vi "Read Device Info.vi"(8 "Error In":errorcluster, 11 "AMS Connection In":T3) -> (0 "Error Out":errorcluster, 1 "Version":T2, 2 "ADS Error":T1 items=["NoError"=0, "InternalError"=1, "NoRTime"=2, "LockedMemoryError"=3, "MailBoxError"=4, "WrongHMsg"=5, "TargetPortNotFound"=6, "TargetMachineNotFound"=7, "UnknownCommandID"=8, "BadTaskID"=9, "NoIO"=10, "UnknownAmsCommand"=11, "Win32Error"=12, "PortNotConnected"=13, "InvalidAmsLength"=14, "InvalidAmsNetID"=15, "AmsSyncAmsError"=22, "AmsSyncNoIndexMap"=23, "InvalidAmsPort"=24, "NoMemory"=25, "TCPSendError"=26, "HostUnreachable"=27, "NoLockedMemory"=1280, "MailboxFull"=1282, "DeviceError"=1792, "DeviceServiceNotSupported"=1793, "DeviceInvalidGroup"=1794, "DeviceInvalidOffset"=1795, "DeviceInvalidAccess"=1796, "DeviceInvalidSize"=1797, "DeviceInvalidData"=1798, "DeviceNotReady"=1799, "DeviceBusy"=1800, "DeviceInvalidContext"=1801, "DeviceNoMemory"=1802, "DeviceInvalidParam"=1803, "DeviceNotFound"=1804, "DeviceSyntaxError"=1805, "DeviceIncompatible"=1806, "DeviceExists"=1807, "DeviceSymboldNotFound"=1808, "DeviceSymbolVersionInvalid"=1809, "DeviceInvalidState"=1810, "DeviceTransModeNotSupported"=1811, "DeviceNotifyHandleInvalid"=1812, "DeviceClientUnknown"=1813, "DeviceNoMoreHandles"=1814, "DeviceInvalidWatchsize"=1815, "DeviceNotInitialized"=1816, "DeviceTimeOut"=1817, "DeviceNoInterface"=1818, "DeviceInvalidInterface"=1819, "DeviceInvalidCLSID"=1820, "DeviceInvalidObjectID"=1821, "ClientError"=1856, "ClientInvalidParameter"=1857, "ClientListEmpty"=1858, "ClientVariableInUse"=1859, "ClientDuplicateInvokeID"=1860, "ClientSyncTimeOut"=1861, "ClientW32OR"=1862, "ClientTimeoutInvalid"=1863, "ClientPortNotOpen"=1864, "ClientNoAmsAddr"=1865, "ClientSyncInternal"=1872, "ClientAddHash"=1873, "ClientRemoveHash"=1874, "ClientNoMoreSymbols"=1875, "ClientSyncResInvalid"=1876, "ClientSyncPortLocked"=1877, "ClientQueueFull"=1878], 3 "Device Name":string)   [LabVIEW 2016, in "TwinCAT ADS.lvlib"]
uses:
  TwinCAT ADS.lvlib
  Low Level/TypeDefs/AMS Connection.ctl
  Low Level/TypeDefs/AMS.ctl
  Low Level/TypeDefs/Device Version.ctl
  Low Level/TypeDefs/ADS Error.ctl
  Low Level/TypeDefs/Command Id.ctl
  Low Level/TypeDefs/State Flag.ctl
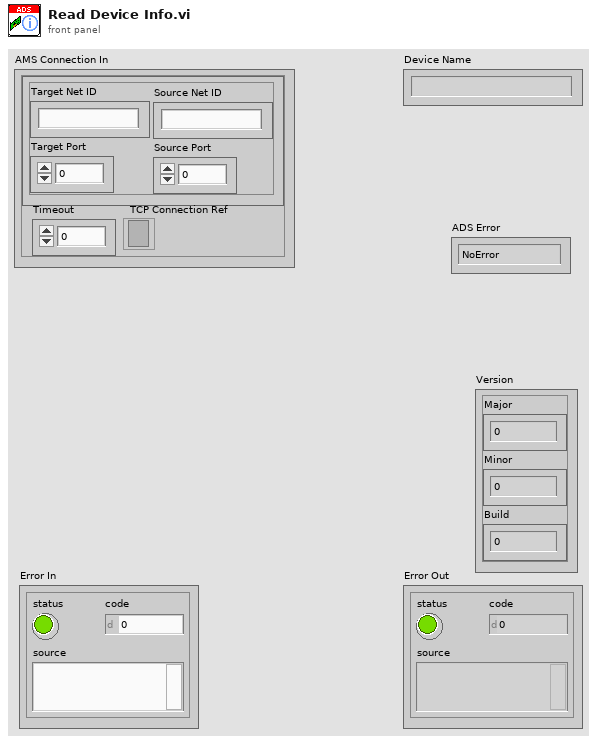
[diagram p1: front panel]
types:
  T1 = typedef "TwinCAT ADS.lvlib/ADS Error.ctl" = u32
  T2 = typedef "TwinCAT ADS.lvlib/Device Version.ctl" = cluster{"Major":u8, "Minor":u8, "Build":u16}
  T3 = typedef "TwinCAT ADS.lvlib/AMS Connection.ctl" = cluster{"AMS":T4, "Timeout":i32, "TCP Connection Ref":refnum<k5>}
  T4 = typedef "TwinCAT ADS.lvlib/AMS.ctl" = cluster{"Target Net ID":string, "Target Port":u16, "Source Net ID":string, "Source Port":u16}
  T5 = enum16{"Standard", "Buffered", "CRLF", "Immediate"}
  T6 = typedef "TwinCAT ADS.lvlib/State Flag.ctl" = u16
  T7 = typedef "TwinCAT ADS.lvlib/Command Id.ctl" = enum16{"Invalid", "ADS Read Device Info", "ADS Read", "ADS Write", "ADS Read State", "ADS Write Control", "ADS Add Device Notification", "ADS Delete Device Notification", "ADS Device Notification", "ADS Read Write"}
  T8 = cluster{"Major Version":u8, "Minor Version":u8, "Build Number":u16}
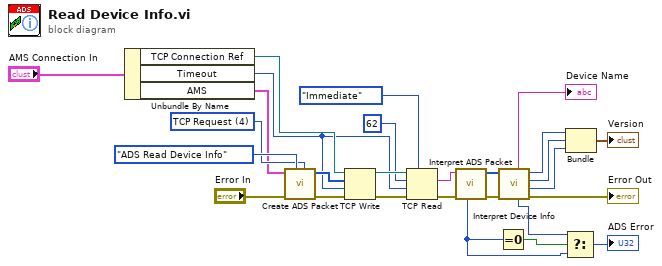
[diagram p0: block diagram]
diagram:
  w26 = T6 4 items=["TCP Request"=4, "TCP Response"=5, "UDP Request"=68, "UDP Respone"=69] ("State Flag")
  n1 = Unbundle By Name("AMS Connection In") -> ("TCP Connection Ref"=w3:refnum<k5>, "Timeout"=w2:i32, "AMS"=w4:T4)
  n2 = call "Create ADS Packet.vi"("State Flag"=w26, "Command ID"=Command_Id."ADS Read Device Info", "Error In"="Error In", "AMS"=w4) -> ("Error Out"=w23:errorcluster, "ADS Packet"=w25:u8[])  [unwired: 6 in]
  n3 = TCP Write(connection ID=w3, data in=w25, error in (no error)=w23, 9:w2) -> (connection ID out=w24:refnum<k5>, error out=w22:errorcluster)  [unwired: 1 out]
  n4 = TCP Read(connection ID=w24, bytes to read=62, error in (no error)=w22, 7:T5."Immediate" ("mode (standard)"), 9:w2) -> (data out=w9:string, error out=w11:errorcluster)  [unwired: 1 out]
  n5 = call "Interpret ADS Packet.vi"("Error In"=w11, "ADS Packet"=w9) -> ("Error Out"=w10:errorcluster, "Data"=w12:u8[], "ADS Error"=w6:T1)  [unwired: 3 in, 4 out]
  n6 = Equal To 0?(x=w6) -> (x = 0?=w8:bool)
  n7 = call "Interpret Device Info.vi"("Error In"=w10, "Data In"=w12) -> ("Error Out"=→"Error Out":errorcluster, "Build Number"=w17:u16, "Minor Version"=w18:u8, "Major Version"=w19:u8, "ADS Error"=w7:T1, "Device Name"=→"Device Name":string)  [unwired: 4 in]
  n8 = Select(t=w7, s=w8, f=w6) -> (s? t:f=→"ADS Error":T1)
  n9 = Bundle("Major Version"=w19, "Minor Version"=w18, "Build Number"=w17) -> (→"Version":T8)  [unwired: 1 in]
